vi "CC FITS Write Filter Names.vi"(8 "error in (no error)":errorcluster, 11 "gfits refnum":T1) -> (0 "error out":errorcluster, 3 "dup gfits refnum":T1)   [LabVIEW 2024]
uses:
  gfitsio/gfitsio-refnum.ctl
  Logging/CC enum Current Values Action.ctl
  gfitsio/gfitsio-write-key-string.vi
  hk-channel-class/hk-channel-class/HK Table/HK Table.lvclass
  gfitsio/gfitsio.lvlib
  Filter Wheel/Filter Wheel Object/Filter Wheel.lvclass
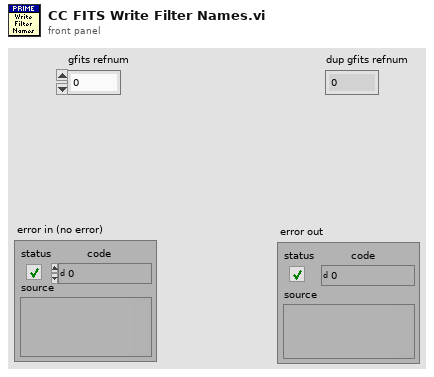
[diagram p1: front panel]
types:
  T1 = typedef "gfitsio.lvlib/gfitsio-refnum.ctl" = u64
  T2 = typedef "CC enum Current Values Action.ctl" = enum16{"Init", "Write Item", "Write Array", "Read Item", "Read Array", "Read All", "Add Channels", "New File", "Add Message", "Get Current Values", "Close"}
  T3 = typedef "Filter Wheel.lvclass/Filter Wheel configuration.ctl" = cluster{"Num Wheels":i32, "Filters":T4[], "Invalid Combinations":i32[][], "Addr":refnum<visa-resource-name>, "Name":string, "Simulate":bool, "Homing Parameters":T5, "Default Speed":u16}
  T4 = typedef "Filter Wheel.lvclass/Filter Wheel Details.ctl" = cluster{"Names":string[], "Relative Position":i32[], "Wheel Name":string}
  T5 = typedef "Filter Wheel Arduino Homing cluster.ctl" = cluster{"Direction (F: CW)":bool, "Speed":i32, "Accel":i32, "Min Distance":i32, "Short Leg":i32, "Error Cnts":i32}
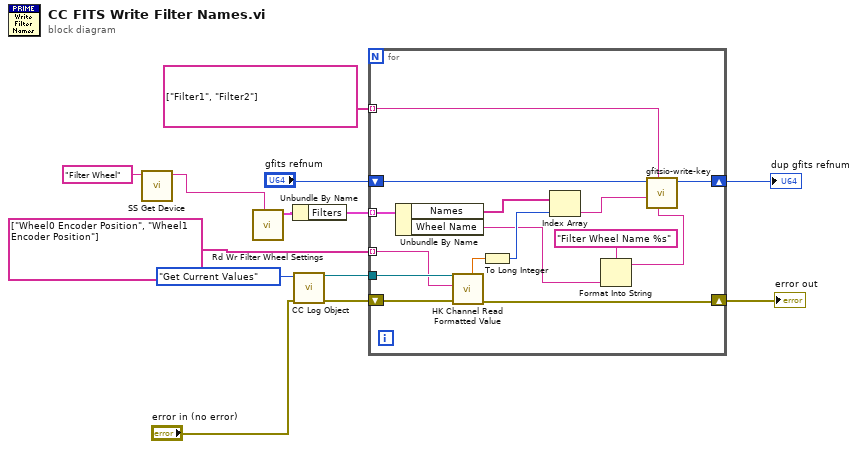
[diagram p0: block diagram]
diagram:
  n1 = call "SS Get Device.vi"("Device Type"="Filter Wheel") -> ("Device Name"=w1:string)  [unwired: 9 in, 1 out]
  n2 = call "Rd Wr Filter Wheel Settings.vi"("Wheel Name"=w1) -> ("Filter Wheel Settings"=w5:T3)  [unwired: 9 in, 1 out]
  n3 = Unbundle By Name(w5) -> ("Filters"=w4:T4[])
  n4 = call "CC Log Object.vi"("error in (no error)"="error in (no error)", "Action"=CC_enum_Current_Values_Action."Get Current Values") -> ("error out"=w8:errorcluster, "HK Channel out"=w12:refnum<class "HK Table.lvclass">)  [unwired: 7 in, 1 out]
  n5 = for {
    tunnel: w12 -> [w28]
    shift-right: [w26] -> w10
    shift-left: "gfits refnum" -> [w27]
    shift-right: [w24] -> w7
    shift-left: w8 -> [w25]
    tunnel: string[] ["Wheel0 Encoder Position", "Wheel1 Encoder Position"] -> [w23] mode=indexing
    tunnel: w4 -> [w21] mode=indexing
    tunnel: string[] ["Filter1", "Filter2"] -> [w17] mode=indexing
    n6 = Unbundle By Name(w21) -> ("Names"=w20:string[], "Wheel Name"=w15:string)
    n7 = call-dynamic "HK Channel Read Formatted Value.vi"("error in (no error)"=w25, "Name"=w23, "HK Table.lvclass"=w28) -> ("error out"=w24:errorcluster, "Value"=w22:dbl)  [unwired: 1 in, 6 out]
    n8 = To Long Integer(number=w22) -> (32bit integer=w19:i32)
    n9 = Index Array(array=w20, index=w19) -> (element=w18:string)
    n10 = Format Into String(format string="Filter Wheel Name %s", w15) -> (resulting string=w14:string)  [unwired: 2 in, 1 out]
    n11 = call-poly "gfitsio-write-key.vi"("comment"=w14, "keyname"=w17, "value"=w18, "gfits refnum"=w27) -> ("dup gfits refnum"=w26:T1)  [unwired: 6 in, 1 out]
  }
  "error out" <- w7
  "dup gfits refnum" <- w10
